vi "Read InputData.vi"(11 "ILC in":refnum<class "ILC.lvclass">) -> (2 "InputData":T1, 3 "ILC out":refnum<class "ILC.lvclass">)   [LabVIEW 2015, in "ILCCommon.lvlib" / "ILC.lvclass"]
uses:
  <userlib>/Common/ILC/ILC/ILC.lvclass
  <userlib>/Common/ILC/Typedefs/Inputs.ctl
  <userlib>/Common/ILC/Configuration/Input Channels.ctl
  <userlib>/Common/ILC/Typedefs/Limit Switches.ctl
  <userlib>/Common/ILC/Typedefs/ADC Raw.ctl
  <userlib>/Common/ILC/ILC/ILC.lvclass/ILC.ctl
  <userlib>/Common/ILC/Typedefs/ILCTypedefs.lvlib
  <userlib>/Common/ILC/Configuration/ILCConfiguration.lvlib
panel:
  # "Limit Switches"
  # "ADCs Raw"
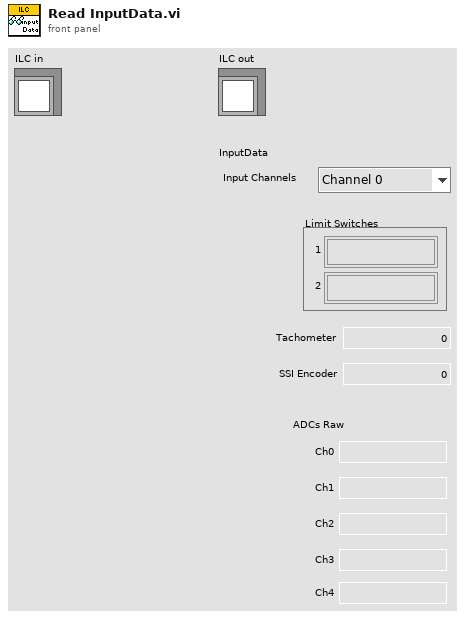
[diagram p1: front panel]
types:
  T1 = typedef "ILCCommon.lvlib/ILCTypedefs.lvlib/Inputs.ctl" = cluster{"Input Channels":T2, "Limit Switches":T3, "Tachometer":u16, "SSI Encoder":i32, "ADC":T4}
  T2 = typedef "ILCCommon.lvlib/ILCConfiguration.lvlib/Input Channels.ctl" = enum16{"Channel 0", "3 Channels", "5 Channels"}
  T3 = typedef "ILCCommon.lvlib/ILCTypedefs.lvlib/Limit Switches.ctl" = cluster{"1":bool, "2":bool}
  T4 = typedef "ILCCommon.lvlib/ILCTypedefs.lvlib/ADC Raw.ctl" = cluster{"Ch0":i32, "Ch1":i32, "Ch2":i32, "Ch3":i32, "Ch4":i32}
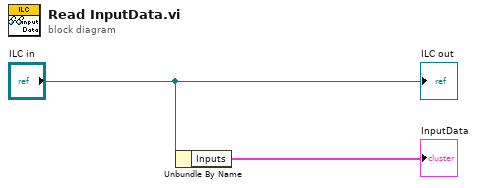
[diagram p0: block diagram]
diagram:
  n1 = Unbundle By Name("ILC in") -> ("Inputs"=→"InputData":T1)
  "ILC out" <- "ILC in"
